vi "AH25_Main.vi"() -> ()   [LabVIEW 2021]
uses:
  GEN_States.ctl
  1375486a-d526-4950-a4e9-ede105372d37.vi
  Sources/Config_Cluster.ctl
  Sources/Data_Cluster.ctl
  <vilib>/Utility/config.llb/NI_LVConfig.lvlib
  Sources/Mode_Enum.ctl
  Sources/Measurement_Cluster.ctl
  Sources/Plotting-Axis.ctl
panel:
  in  "Control Tab":enum32{"General", "Configs"}(tab)
  out "Oven Warning":bool
  out "Capacitance":dbl
  in  "StopM_Button":bool
  in  "Log_Button":bool
  in  "Measure_Button":bool
  out "Globals":bool
  out "AH 2500A":bool
  out "Logging":bool
  out "Measuring":bool
  out "Magnetic Field":dbl
  out "Temperature":dbl
  in  "LoadConfig_Button":bool
  in  "ApplyConfig_Button":bool
  in  "Measure rate (1/s)":i32
  in  "SaveConfig_Button":bool
  in  "Retry_Button":bool
  in  "Config Path (Blank is default)":path
  in  "AH2500 VISA COM":refnum<visa-resource-name>
  in  "Global Temp VAR":refnum<k21>
  in  "Global Mag VAR":refnum<k21>
  in  "Logging Path":path
  in  "Display Tab":enum32{"Program Monitor", "Test Plot"}(tab)
  out "Status":string
  in  "Clear_Button":bool
  in  "Y-Axis":T1
  in  "X-Axis":T1
  out "Test Graph":cluster{"X":dbl, "Y":dbl}[](graph)
  in  "Max Elements":i32=5000
  in  "Exit_Button":bool
  # "Instrument Settings"
  # "Global Var. Settings"
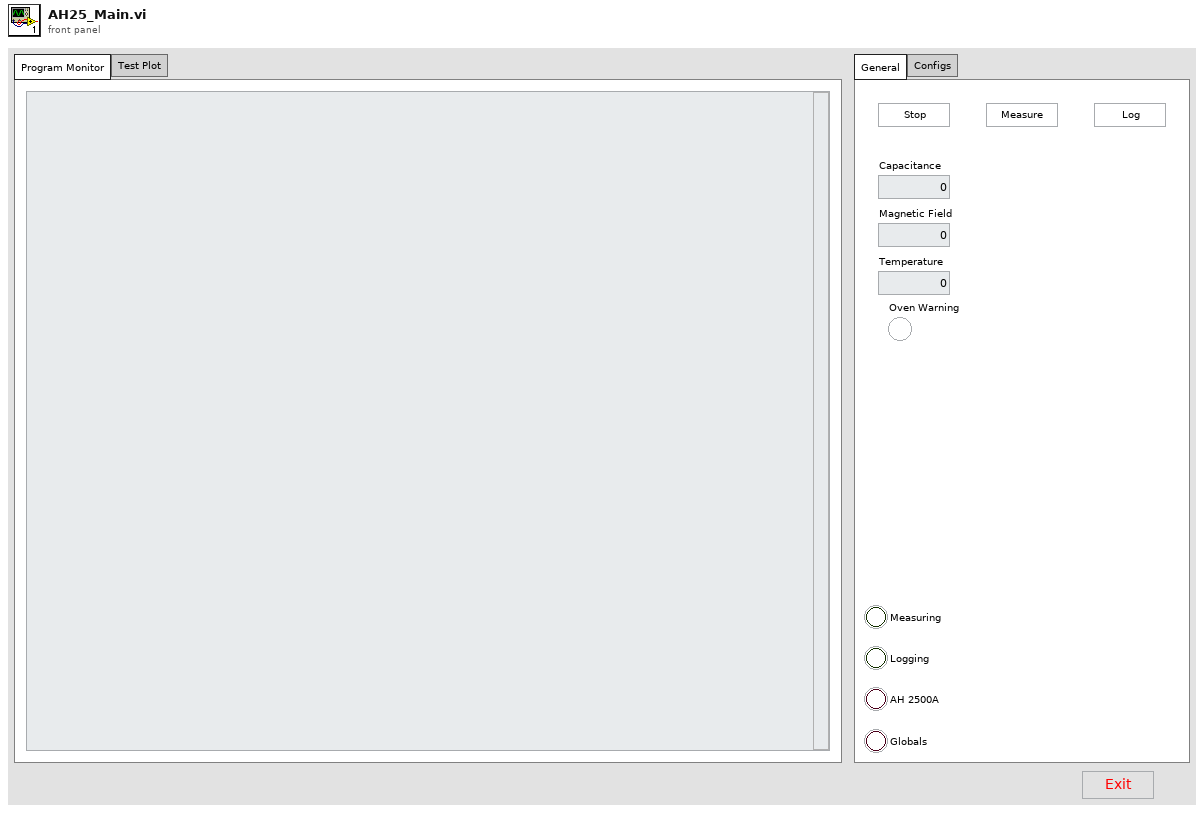
[diagram p1: front panel]
types:
  T1 = typedef "Plotting-Axis.ctl" = enum16{"Time", "Temperature", "MagneticField", "Primary", "Secondary"}
  T2 = typedef "GEN_States.ctl" = enum16{"ClearBuffers", "SwitchToMeas", "SwitchToLog", "SwitchToOff", "Disconnect", "ApplyConfig", "ExitSafe", "RefreshPlotMUnits", "UpdatePlots", "RefreshMUnits", "ChangeOperation", "Read/WriteAll", "RetryComs", "SendProfile", "InitGUI", "RefreshGUI", "ComsFail", "SaveConfig", "Idle", "ProgInit"}
  T3 = typedef "Data_Cluster.ctl" = cluster{"Value":dbl, "GUI Data Cluster":cluster{"SBR":u8}, "Timing":cluster{"Last Operation":dbl}, "Measurements":T4[]}
  T4 = typedef "Measurement_Cluster.ctl" = cluster{"Time Stamp":timestamp, "Cap":dbl, "Temperature":dbl, "MagneticField":dbl}
  T5 = typedef "Config_Cluster.ctl" = cluster{"General":cluster{"Config.ini":path, "Default Logging Path":path}, "Hardware":cluster{"AHC VISA COM":refnum<visa-resource-name>, "Measure Rate (1/s)":i32, "Global T VAR":refnum<k21>, "Global B VAR":refnum<k21>}, "Operation":cluster{"Operation Mode":T6, "Status":string, "NewLog?":bool}}
  T6 = typedef "Mode_Enum.ctl" = enum16{"Logging", "Idle-Off", "Idle"}
  T7 = enum8{"Enabled", "Disabled", "Disabled and Grayed Out"}
  T8 = typedef "NI_LVConfig.lvlib/Config Data RefNum.ctl" = refnum<k1>
  T9 = cluster{"Logging Path":path, "AH2500 VISA COM":refnum<visa-resource-name>, "Measure rate (1/s)":i32, "Global Temp VAR":refnum<k21>, "Global Mag VAR":refnum<k21>}
  T10 = cluster{"Primary Measurement":dbl, "Secondary Measurement":dbl, "T Var":dbl, "B Var":dbl}
  T11 = typedef "GEN_States.ctl" = enum16{"ClearBuffers", "SwitchToMeas", "SwitchToLog", "SwitchToOff", "Disconnect", "ApplyConfig", "ExitSafe", "RefreshPlotMUnits", "UpdatePlots", "RefreshMUnits", "ChangeOperation", "Read/WriteAll", "RetryComs", "SendProfile", "InitGUI", "RefreshGUI", "ComsFail", "LoadProfile", "SaveProfile", "SaveConfig", "Idle", "ProgInit"}
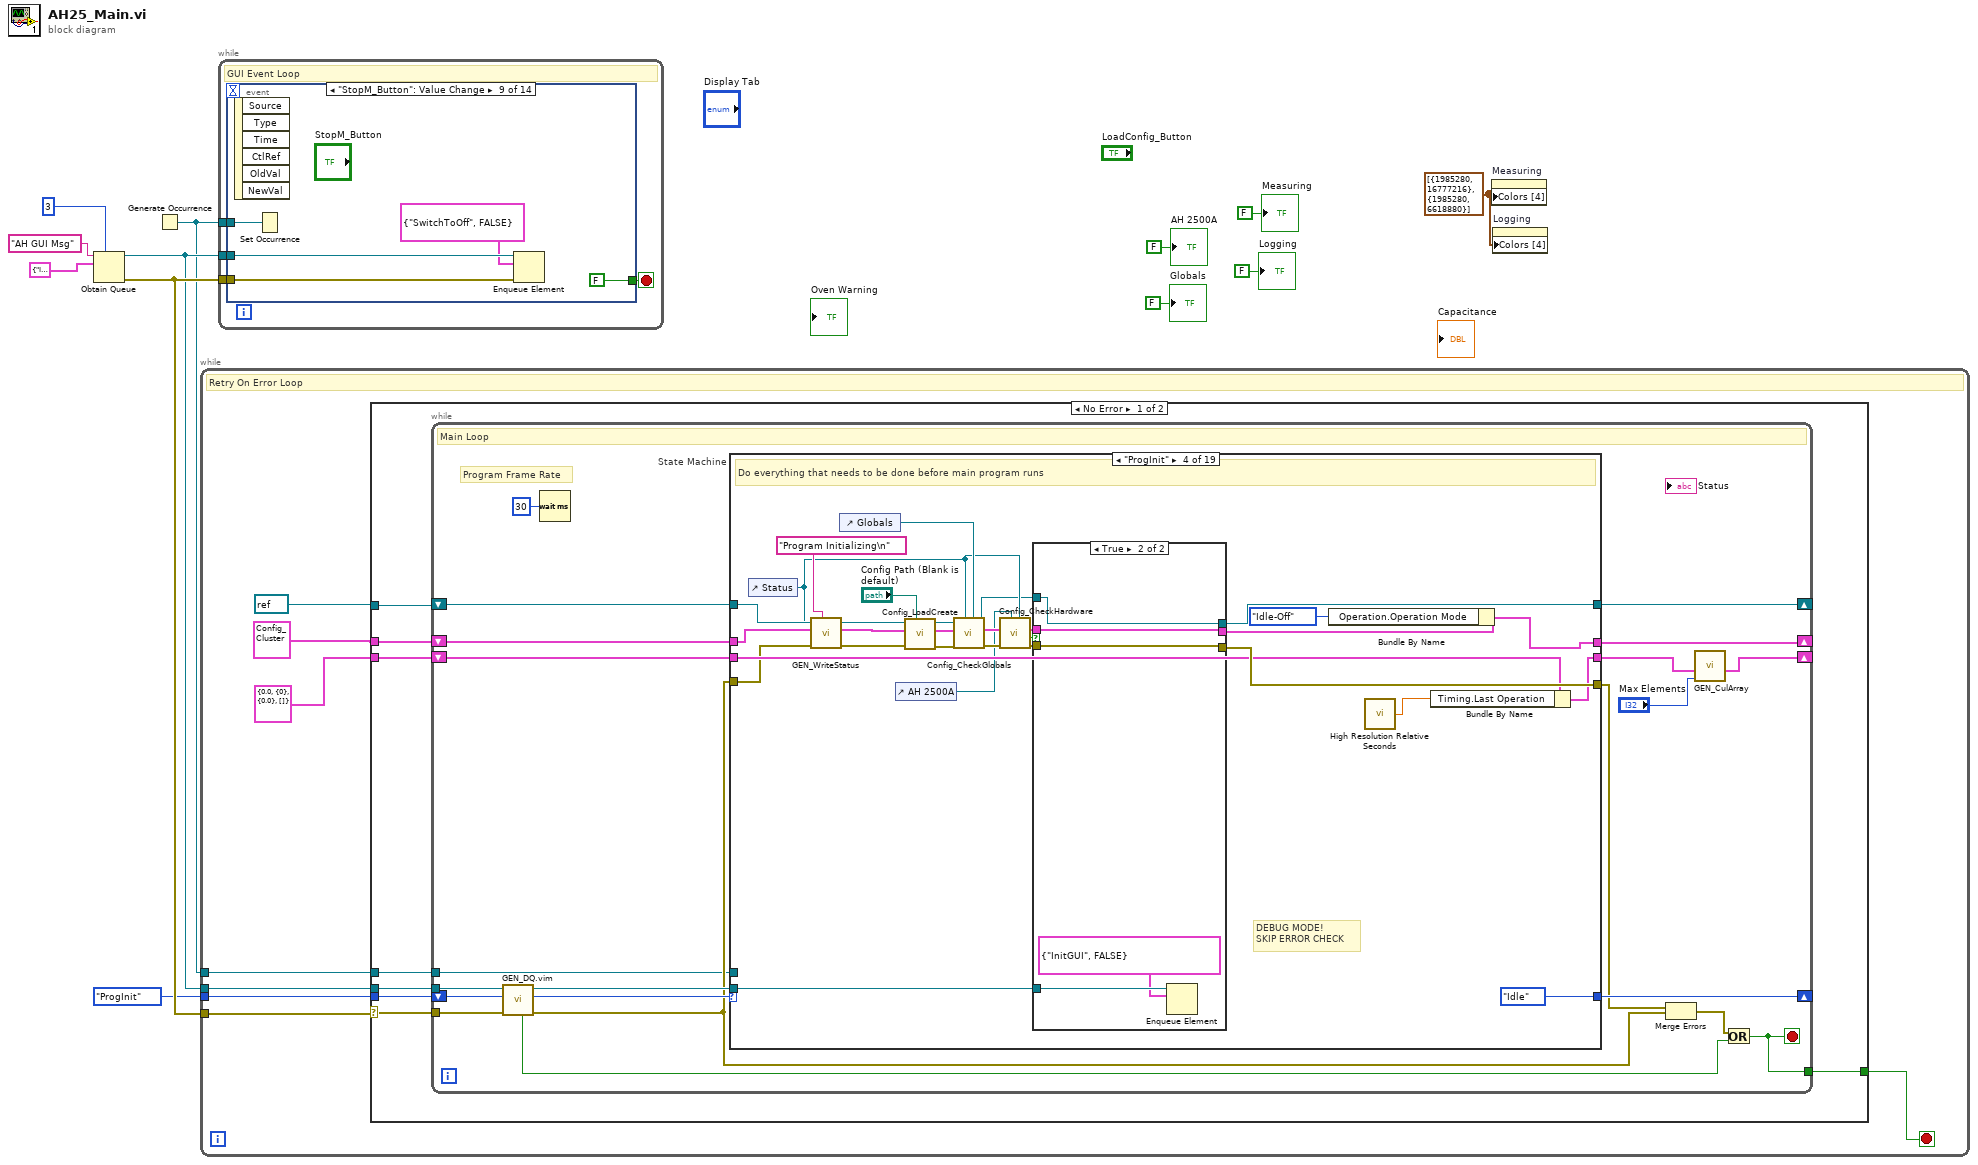
[diagram p0: block diagram]
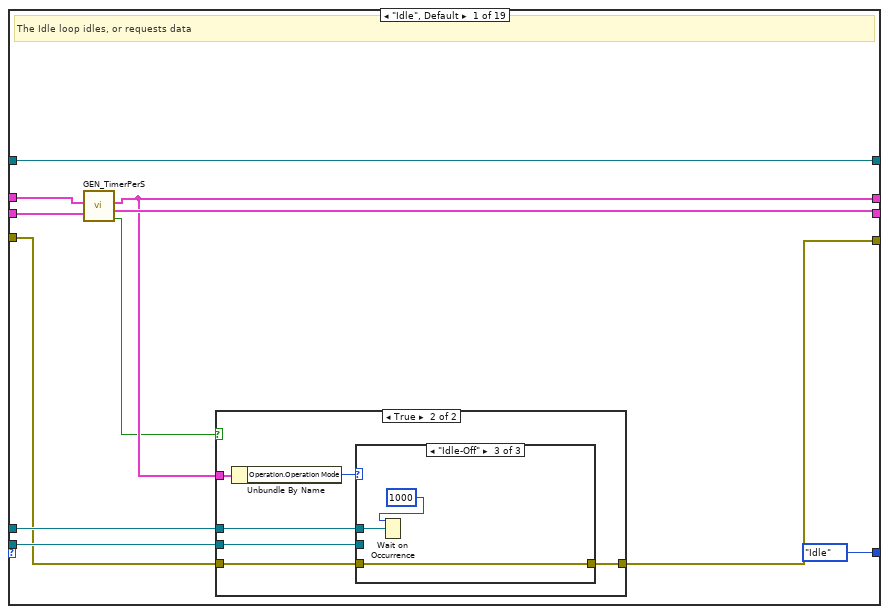
[diagram p2: hidden frame]
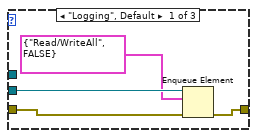
[diagram p4: hidden frame]
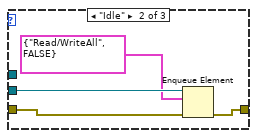
[diagram p5: hidden frame]
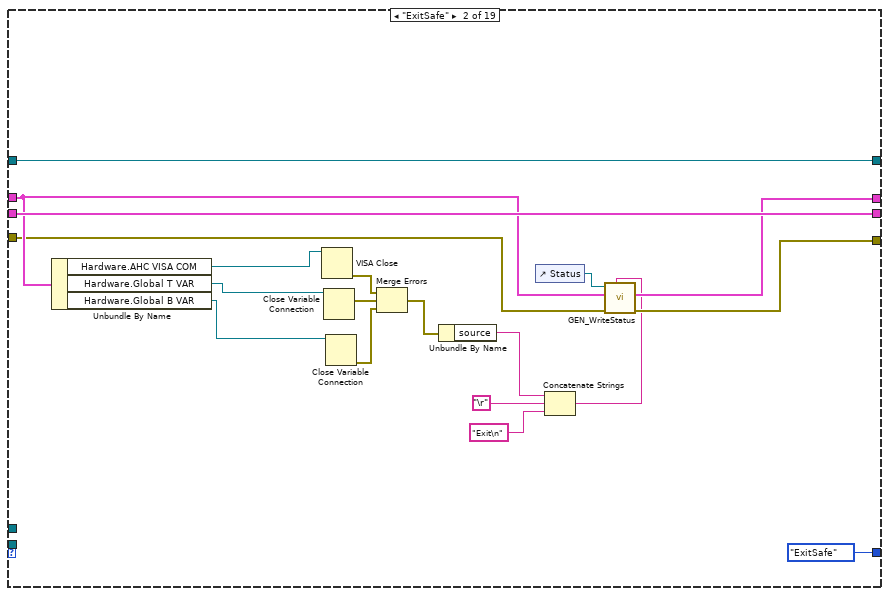
[diagram p6: hidden frame]
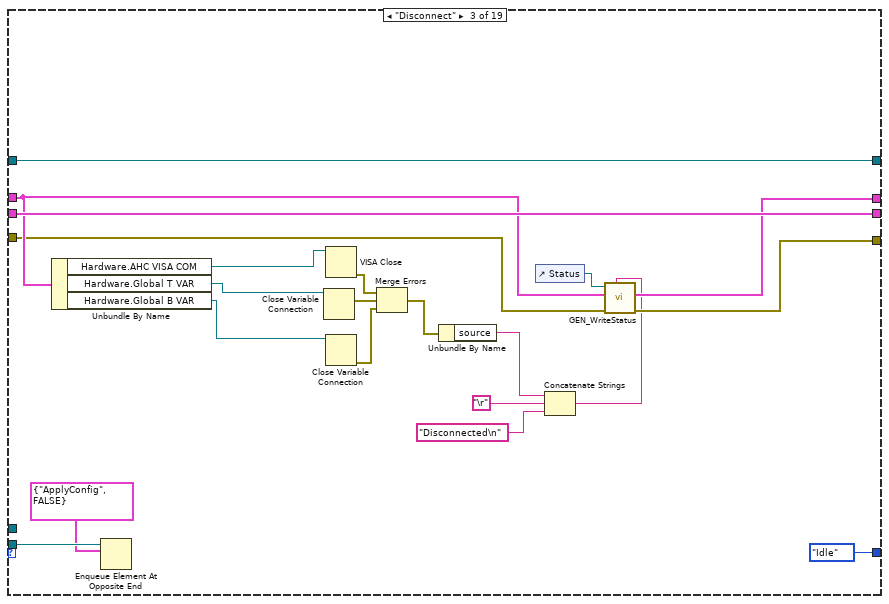
[diagram p7: hidden frame]
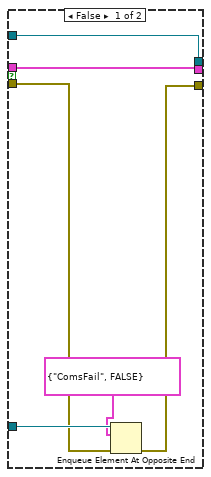
[diagram p8: hidden frame]
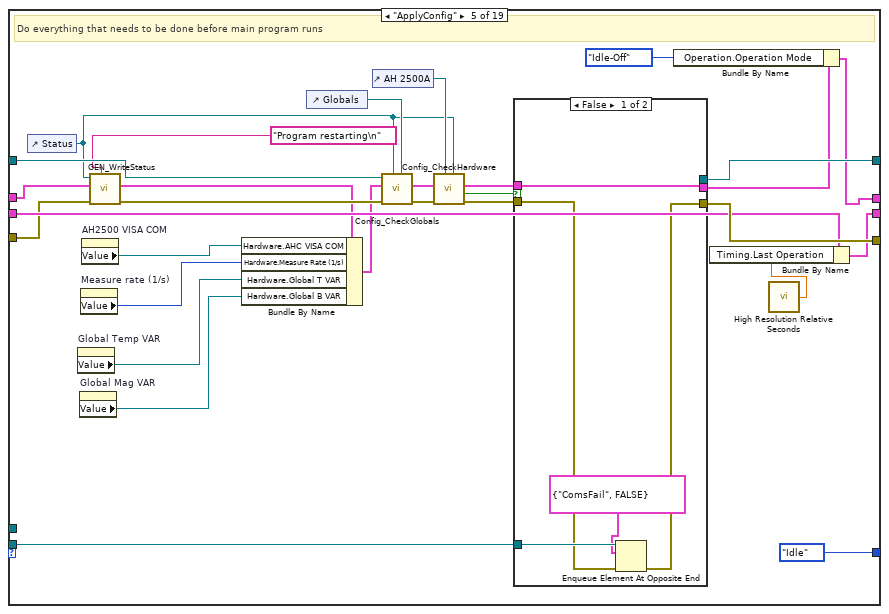
[diagram p9: hidden frame]
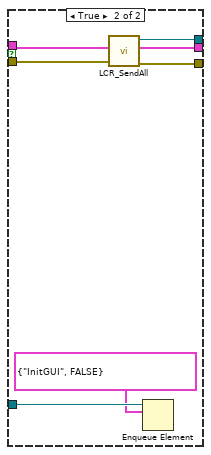
[diagram p10: hidden frame]
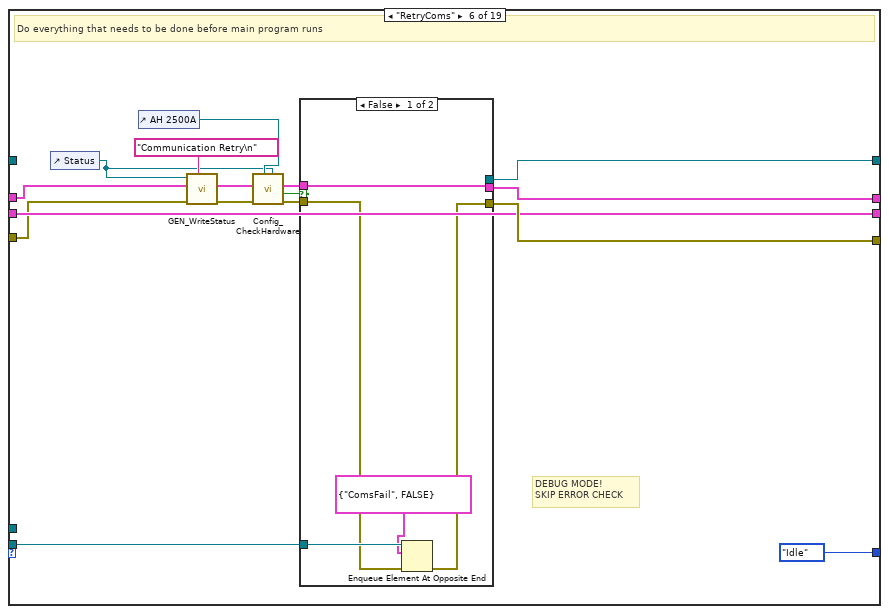
[diagram p11: hidden frame]
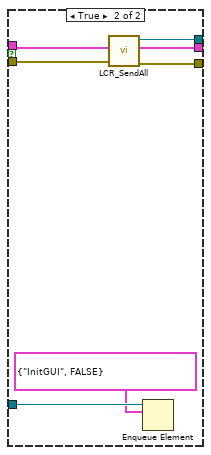
[diagram p12: hidden frame]
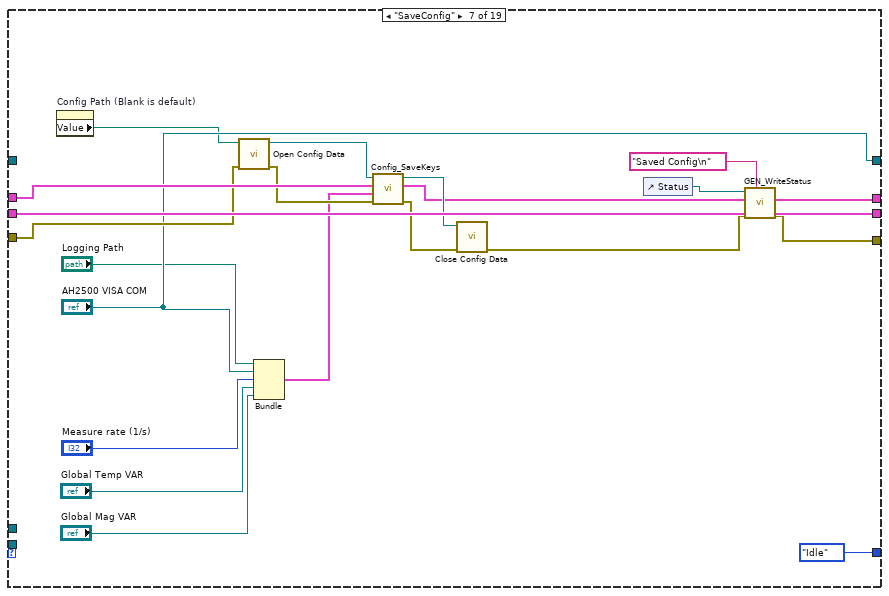
[diagram p13: hidden frame]
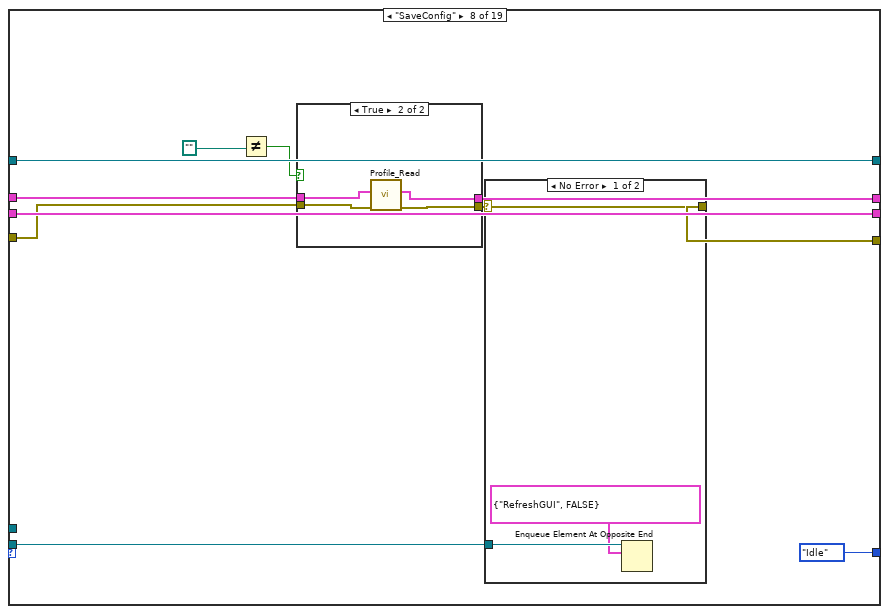
[diagram p14: hidden frame]
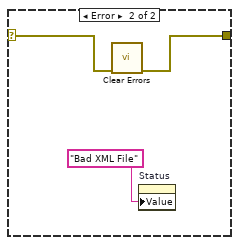
[diagram p15: hidden frame]
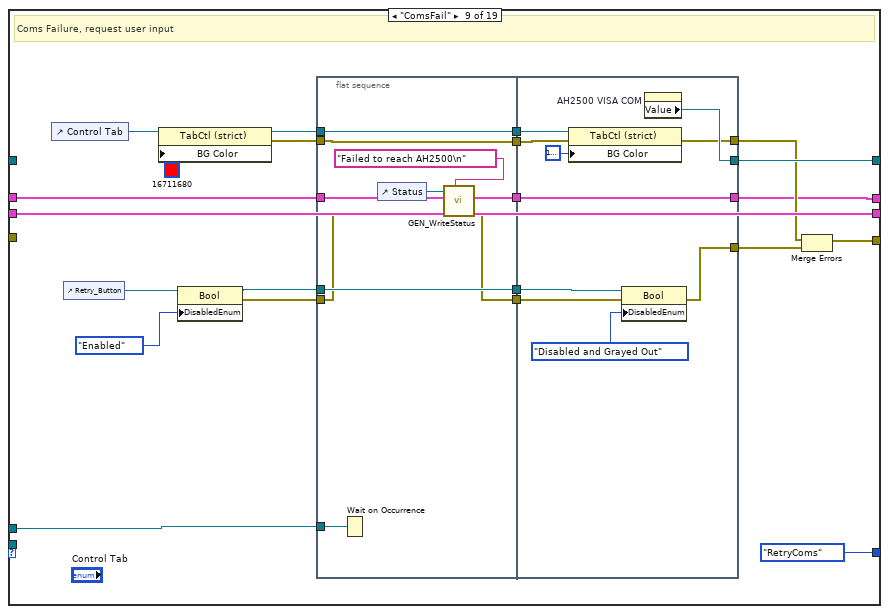
[diagram p17: hidden frame]
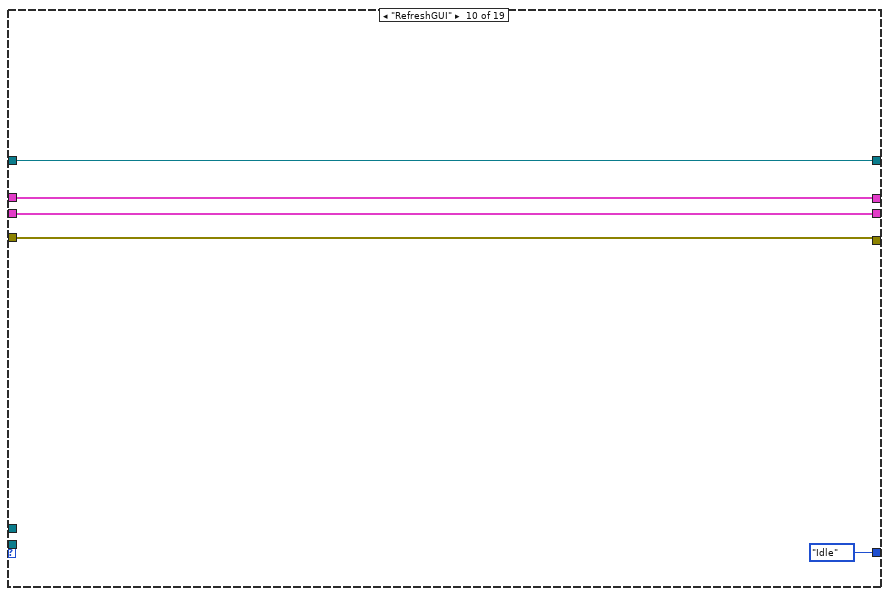
[diagram p18: hidden frame]
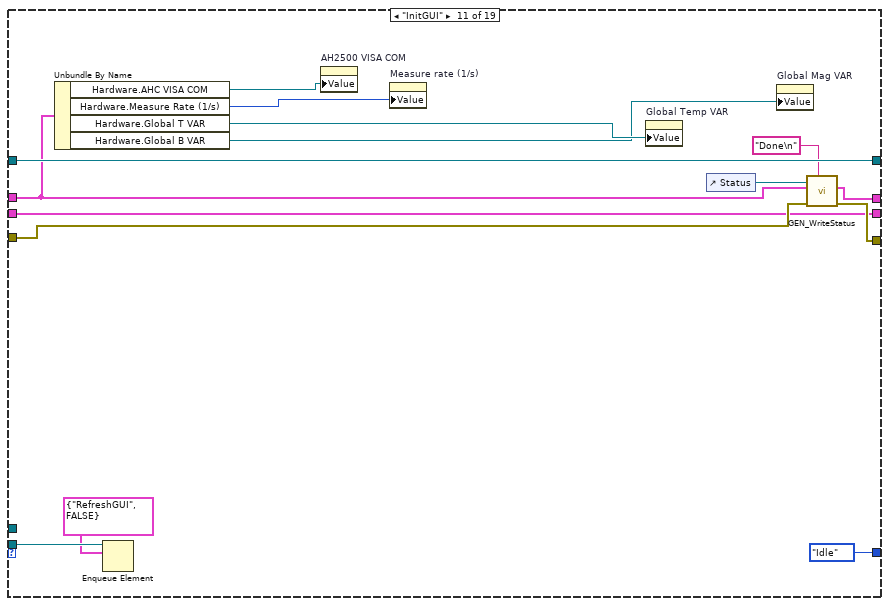
[diagram p19: hidden frame]
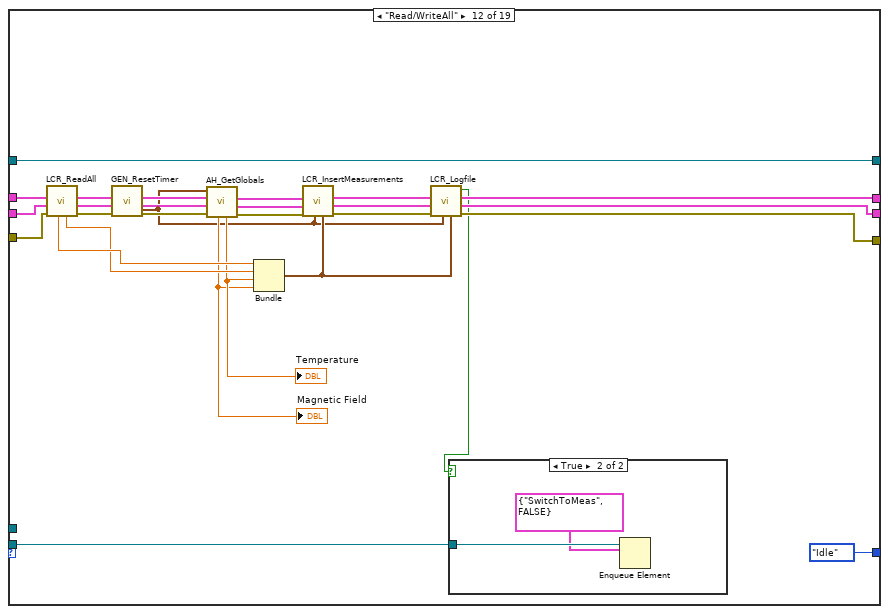
[diagram p20: hidden frame]
diagram:
  w1 = cluster{u32, u32}[] [{1985280, 16777216}, {1985280, 6618880}] ("Colors [4]")
  n1 = Obtain Queue(max queue size (-1, unlimited)=3, name (unnamed)="AH GUI Msg", element data type=cluster{T2, bool} {enum."Idle", TRUE}) -> (queue out=w8:refnum<queue>, error out=w9:errorcluster)  [unwired: 2 in, 1 out]
  n2 = Generate Occurrence() -> (w6:refnum<k4>)
  n3 = while {
    tunnel: w9 -> [w20]
    tunnel: w8 -> [w19]
    tunnel: GEN_States."ProgInit" ("State") -> [w18]
    tunnel: w6 -> [w13]
    stop <- w17 stop-if-true
    # "Retry On Error Loop"
    n4 = case shown="No Error" w20 {
      selector: w20 -> [w28 _]
      tunnel: w19 -> [w27 _]
      tunnel: w18 -> [w26 _]
      tunnel: [w25 TRUE] -> w17
      tunnel: refnum<visa-resource-name> refnum ("LCR VISA COM") -> [w24 _]
      tunnel: T5 {"General"={"Config.ini"=path "", "Default Logging Path"=path ""}, "Hardware"={"AHC VISA COM"="", "Measure Rate (1/s)"=0, "Global T VAR"="", "Global B VAR"=""}, "Operation"={"Operation Mode"=enum."Logging", "Status"="", "NewLog?"=FALSE}} -> [w23 _]
      tunnel: T3 {"Value"=0.0, "GUI Data Cluster"={"SBR"=0}, "Timing"={"Last Operation"=0.0}, "Measurements"=[]} -> [w22 _]
      tunnel: w13 -> [w21 _]
      frame No Error {
        n5 = while {
          tunnel: w28 -> [w48]
          tunnel: w27 -> [w47]
          shift-right: [w40] -> _
          shift-left: w26 -> [w46]
          tunnel: [w42] -> w25
          shift-right: [w39] -> _
          shift-left: w24 -> [w41]
          shift-right: [w36] -> _
          shift-left: w23 -> [w37]
          shift-right: [w30] -> _
          shift-left: w22 -> [w35]
          tunnel: w21 -> [w32]
          stop <- w42 stop-if-true
          # "Program Frame Rate"
          # "Main Loop"
          n6 = call "GEN_DQ.vim"("error in (no error)"=w48, "Variant"=w46, "queue In"=w47) -> ("error out"=w34:errorcluster, "Variant Out"=w45:T2, "queue out"=w38:refnum<queue>, "Exit?"=w43:bool)  [unwired: 5 in]
          n7 = Wait (ms)(milliseconds to wait=u32 30) -> ()  [unwired: 1 out]
          n8 = case "State Machine" shown="\"ProgInit\"" w45 {
            tunnel: w41 -> [w60 w97 w118 w145 w186 _ _ w259 _ w317 w333 w361 w380 w398 w424 w443 w451 w459 w465]
            tunnel: [GEN_States."Idle" ("State") GEN_States."ExitSafe" ("State") GEN_States."Idle" ("State") GEN_States."Idle" ("State") GEN_States."Idle" ("State") GEN_States."Idle" ("State") GEN_States."Idle" ("State") GEN_States."Idle" ("State") GEN_States."RetryComs" ("State") GEN_States."Idle" ("State") GEN_States."Idle" ("State") GEN_States."Idle" ("State") GEN_States."Idle" ("State") GEN_States."Idle" ("State") w410 GEN_States."Idle" ("State") GEN_States."Idle" ("State") GEN_States."Idle" ("State") GEN_States."Idle" ("State")] -> w40
            tunnel: [w60 w97 w118 w140 w181 w209 "AH2500 VISA COM" w259 w286 w317 w333 w361 w380 w398 w424 w443 w451 w459 w465] -> w39
            tunnel: w38 -> [w57 _ w102 w139 w180 w208 _ w249 _ _ w331 w334 _ _ _ _ _ _ _]
            tunnel: w37 -> [w54 w91 w113 w131 w172 w206 w245 w255 w274 w314 w327 w360 w378 w396 w422 w442 w448 w456 w464]
            tunnel: [w51 w90 w112 w132 w173 w210 w235 w254 w273 w314 w326 w355 w375 w393 w411 w442 w448 w456 w464] -> w36
            tunnel: w35 -> [w53 w96 w117 w138 w179 w207 w248 w258 w288 w315 w319 w352 w379 w397 w423 w438 w449 w457 w462]
            tunnel: [w52 w96 w117 w137 w178 w207 w248 w258 w288 w315 w319 w349 w379 w397 w423 w437 w449 w457 w461] -> w31
            tunnel: w34 -> [w56 w89 w111 w129 w171 w203 w244 w256 _ w316 w324 w359 w370 w388 w416 w436 w447 w455 w463]
            tunnel: [w55 w88 w110 w141 w182 w211 w231 w250 w277 w316 w323 w356 w369 w387 w415 w436 w447 w455 w463] -> w33
            tunnel: w32 -> [w58 _ _ _ _ _ _ _ w287 _ _ _ _ _ _ _ _ _ _]
            frame "Idle", Default {
              # "The Idle loop idles, or requests data"
              n9 = call "GEN_TimerPerS.vi"("Data_In"=w53, "Config_In"=w54) -> ("Time"=w50:bool, "Data_In 2"=w52:T3, "Config_In 2"=w51:T5)  [unwired: 7 in]
              n10 = case shown="True" w50 {
                tunnel: w58 -> [_ w66]
                tunnel: w57 -> [_ w65]
                tunnel: w56 -> [w61 w64]
                tunnel: [w61 w63] -> w55
                tunnel: w51 -> [_ w62]
                frame False {
                }
                frame True {
                  n11 = Unbundle By Name(w62) -> ("Operation.Operation Mode"=w67:T6)
                  n12 = case shown="\"Idle-Off\"" w67 {
                    tunnel: w66 -> [_ _ w78]
                    tunnel: w65 -> [w71 w75 _]
                    tunnel: w64 -> [w70 w74 w77]
                    tunnel: [w68 w72 w77] -> w63
                    frame "Logging", Default {
                      n13 = Enqueue Element(queue=w71, element=cluster{T2, bool} {enum."Read/WriteAll", FALSE}, error in (no error)=w70) -> (error out=w68:errorcluster)  [unwired: 1 in, 2 out]
                    }
                    frame "Idle" {
                      n14 = Enqueue Element(queue=w75, element=cluster{T2, bool} {enum."Read/WriteAll", FALSE}, error in (no error)=w74) -> (error out=w72:errorcluster)  [unwired: 1 in, 2 out]
                    }
                    frame "Idle-Off" {
                      n15 = Wait on Occurrence(2:w78, 3:1000 ("ms timeout (-1)")) -> ()  [unwired: 1 in, 1 out]
                    }
                  }
                }
              }
            }
            frame "ExitSafe" {
              n16 = Unbundle By Name(w91) -> ("Hardware.AHC VISA COM"=w80:refnum<visa-resource-name>, "Hardware.Global T VAR"=w94:refnum<k21>, "Hardware.Global B VAR"=w93:refnum<k21>)
              n17 = VISA Close(VISA resource name=w80) -> (error out=w79:errorcluster)  [unwired: 1 in]
              n18 = Close Variable Connection(11:w94) -> (0:w86:errorcluster)  [unwired: 1 in]
              n19 = Close Variable Connection(11:w93) -> (0:w87:errorcluster)  [unwired: 1 in]
              n20 = Merge Errors(w79, w86, w87) -> (w85:errorcluster)
              n21 = Unbundle By Name(w85) -> ("source"=w83:string)
              n22 = control-ref of="Status"() -> (w92:refnum<vi>)
              n23 = Concatenate Strings(w83, "\r", "Exit\n" ("string")) -> (w84:string)
              n24 = call "GEN_WriteStatus.vi"("Input String"=w84, "error in (no error)"=w89, "Config_Cluster"=w91, "Status Ref"=w92) -> ("error out"=w88:errorcluster, "Config_Cluster Out"=w90:T5)  [unwired: 6 in]
            }
            frame "Disconnect" {
              n25 = Unbundle By Name(w113) -> ("Hardware.AHC VISA COM"=w99:refnum<visa-resource-name>, "Hardware.Global T VAR"=w116:refnum<k21>, "Hardware.Global B VAR"=w115:refnum<k21>)
              n26 = Enqueue Element At Opposite End(queue=w102, element=cluster{T2, bool} {enum."ApplyConfig", FALSE}) -> ()  [unwired: 2 in, 3 out]
              n27 = Close Variable Connection(11:w116) -> (0:w108:errorcluster)  [unwired: 1 in]
              n28 = VISA Close(VISA resource name=w99) -> (error out=w98:errorcluster)  [unwired: 1 in]
              n29 = Close Variable Connection(11:w115) -> (0:w109:errorcluster)  [unwired: 1 in]
              n30 = Merge Errors(w98, w108, w109) -> (w107:errorcluster)
              n31 = Unbundle By Name(w107) -> ("source"=w105:string)
              n32 = control-ref of="Status"() -> (w114:refnum<vi>)
              n33 = Concatenate Strings(w105, "\r", "Disconnected\n" ("string")) -> (w106:string)
              n34 = call "GEN_WriteStatus.vi"("Input String"=w106, "error in (no error)"=w111, "Config_Cluster"=w113, "Status Ref"=w114) -> ("error out"=w110:errorcluster, "Config_Cluster Out"=w112:T5)  [unwired: 6 in]
            }
            frame "ProgInit" {
              # "DEBUG MODE!\nSKIP ERROR CHECK"
              # "Do everything that needs to be done before main program runs"
              n35 = control-ref of="Status"() -> (w120:refnum<vi>)
              n36 = call "GEN_WriteStatus.vi"("Input String"="Program Initializing\n" ("Status"), "error in (no error)"=w129, "Config_Cluster"=w131, "Status Ref"=w120) -> ("error out"=w128:errorcluster, "Config_Cluster Out"=w130:T5)  [unwired: 6 in]
              n37 = control-ref of="Globals"() -> (w122:refnum<vi>)
              n38 = control-ref of="AH 2500A"() -> (w121:refnum<vi>)
              n39 = call "Config_LoadCreate.vi"("Config In"="Config Path (Blank is default)", "error In"=w128, "Configuration Cluster"=w130, "AH VISA COM"=w145) -> ("error out"=w124:errorcluster, "Configuration Cluster Out"=w125:T5, "AHC VISA COM Out"=w127:refnum<visa-resource-name>)  [unwired: 5 in]
              n40 = call "Config_CheckGlobals.vi"("GlobalsLED Ref"=w122, "Status Ref"=w120, "error in (no error)"=w124, "Config Cluster"=w125, "VISA resource name"=w127) -> ("error out"=w123:errorcluster, "Config Cluster Out"=w126:T5, "VISA resource name out"=w119:refnum<visa-resource-name>)  [unwired: 4 in]
              n41 = call "Config_CheckHardware.vi"("Status Ref"=w120, "HM 8119"=w121, "error in (no error)"=w123, "Config Cluster"=w126) -> ("error out"=w143:errorcluster, "Connected?"=w144:bool, "Config Cluster Out"=w142:T5)  [unwired: 5 in]
              n42 = case shown="True" w144 {
                tunnel: w143 -> [w149 w157]
                tunnel: w142 -> [w152 w158]
                tunnel: w119 -> [w153 w154]
                tunnel: [w153 w154] -> w140
                tunnel: [w152 w158] -> w135
                tunnel: [w148 w157] -> w141
                tunnel: w139 -> [w151 w156]
                frame False {
                  n43 = Enqueue Element At Opposite End(queue=w151, element=cluster{T2, bool} {enum."ComsFail", FALSE}, error in (no error)=w149) -> (error out=w148:errorcluster)  [unwired: 1 in, 2 out]
                }
                frame True {
                  n44 = Enqueue Element(queue=w156, element=cluster{T2, bool} {enum."InitGUI", FALSE}) -> ()  [unwired: 2 in, 3 out]
                }
              }
              n45 = Bundle By Name(cluster=w135, "Operation.Operation Mode"=Mode_Enum."Idle-Off") -> (w132:T5)
              n46 = call <vilib>:"High Resolution Relative Seconds.vi"() -> ("relative seconds"=w136:dbl)
              n47 = Bundle By Name(cluster=w138, "Timing.Last Operation"=w136) -> (w137:T3)
            }
            frame "ApplyConfig" {
              # "Do everything that needs to be done before main program runs"
              n48 = control-ref of="Status"() -> (w160:refnum<vi>)
              n49 = property on="Global Temp VAR" class="Variable (strict)"() -> ("Value"=w164:refnum<k21>)  [unwired: 2 in, 2 out]
              n50 = property on="Global Mag VAR" class="Variable (strict)"() -> ("Value"=w163:refnum<k21>)  [unwired: 2 in, 2 out]
              n51 = property on="Measure rate (1/s)" class="DigNum (strict)"() -> ("Value"=w165:i32)  [unwired: 2 in, 2 out]
              n52 = property on="AH2500 VISA COM" class="VISAName"() -> ("Value"=w159:refnum<visa-resource-name>)  [unwired: 2 in, 2 out]
              n53 = call "GEN_WriteStatus.vi"("Input String"="Program restarting\n" ("Status"), "error in (no error)"=w171, "Config_Cluster"=w172, "Status Ref"=w160) -> ("error out"=w170:errorcluster, "Config_Cluster Out"=w167:T5)  [unwired: 6 in]
              n54 = Bundle By Name(cluster=w167, "Hardware.AHC VISA COM"=w159, "Hardware.Measure Rate (1/s)"=w165, "Hardware.Global T VAR"=w164, "Hardware.Global B VAR"=w163) -> (w166:T5)
              n55 = control-ref of="Globals"() -> (w162:refnum<vi>)
              n56 = control-ref of="AH 2500A"() -> (w161:refnum<vi>)
              n57 = call "Config_CheckGlobals.vi"("GlobalsLED Ref"=w162, "Status Ref"=w160, "error in (no error)"=w170, "Config Cluster"=w166, "VISA resource name"=w186) -> ("error out"=w168:errorcluster, "Config Cluster Out"=w169:T5)  [unwired: 4 in, 1 out]
              n58 = call "Config_CheckHardware.vi"("Status Ref"=w160, "HM 8119"=w161, "error in (no error)"=w168, "Config Cluster"=w169) -> ("error out"=w184:errorcluster, "Connected?"=w185:bool, "Config Cluster Out"=w183:T5)  [unwired: 5 in]
              n59 = case shown="False" w185 {
                tunnel: w184 -> [w189 w198]
                tunnel: w183 -> [w192 w199]
                tunnel: [_ w197] -> w181
                tunnel: [w192 w196] -> w176
                tunnel: [w188 w195] -> w182
                tunnel: w180 -> [w191 w194]
                frame False {
                  n60 = Enqueue Element At Opposite End(queue=w191, element=cluster{T2, bool} {enum."ComsFail", FALSE}, error in (no error)=w189) -> (error out=w188:errorcluster)  [unwired: 1 in, 2 out]
                }
                frame True {
                  n61 = call "LCR_SendAll.vi"("error in (no error)"=w198, "Configuration Cluster"=w199) -> ("error out"=w195:errorcluster, "Configuration Cluster Out"=w196:T5, "VISA resource name out"=w197:refnum<visa-resource-name>)  [unwired: 7 in]
                  n62 = Enqueue Element(queue=w194, element=cluster{T2, bool} {enum."InitGUI", FALSE}) -> ()  [unwired: 2 in, 3 out]
                }
              }
              n63 = Bundle By Name(cluster=w176, "Operation.Operation Mode"=Mode_Enum."Idle-Off") -> (w173:T5)
              n64 = call <vilib>:"High Resolution Relative Seconds.vi"() -> ("relative seconds"=w177:dbl)
              n65 = Bundle By Name(cluster=w179, "Timing.Last Operation"=w177) -> (w178:T3)
            }
            frame "RetryComs" {
              # "DEBUG MODE!\nSKIP ERROR CHECK"
              # "Do everything that needs to be done before main program runs"
              n66 = control-ref of="Status"() -> (w200:refnum<vi>)
              n67 = control-ref of="AH 2500A"() -> (w201:refnum<vi>)
              n68 = call "GEN_WriteStatus.vi"("Input String"="Communication Retry\n", "error in (no error)"=w203, "Config_Cluster"=w206, "Status Ref"=w200) -> ("error out"=w202:errorcluster, "Config_Cluster Out"=w205:T5)  [unwired: 6 in]
              n69 = call "Config_CheckHardware.vi"("Status Ref"=w200, "HM 8119"=w201, "error in (no error)"=w202, "Config Cluster"=w205) -> ("error out"=w213:errorcluster, "Connected?"=w214:bool, "Config Cluster Out"=w212:T5)  [unwired: 5 in]
              n70 = case shown="False" w214 {
                tunnel: w213 -> [w217 w226]
                tunnel: w212 -> [w220 w227]
                tunnel: [_ w225] -> w209
                tunnel: [w220 w224] -> w210
                tunnel: [w216 w223] -> w211
                tunnel: w208 -> [w219 w222]
                frame False {
                  n71 = Enqueue Element At Opposite End(queue=w219, element=cluster{T2, bool} {enum."ComsFail", FALSE}, error in (no error)=w217) -> (error out=w216:errorcluster)  [unwired: 1 in, 2 out]
                }
                frame True {
                  n72 = call "LCR_SendAll.vi"("error in (no error)"=w226, "Configuration Cluster"=w227) -> ("error out"=w223:errorcluster, "Configuration Cluster Out"=w224:T5, "VISA resource name out"=w225:refnum<visa-resource-name>)  [unwired: 7 in]
                  n73 = Enqueue Element(queue=w222, element=cluster{T2, bool} {enum."InitGUI", FALSE}) -> ()  [unwired: 2 in, 3 out]
                }
              }
            }
            frame "SaveConfig" {
              n74 = property on="Config Path (Blank is default)" class="Path"() -> ("Value"=w238:path)  [unwired: 2 in, 2 out]
              n75 = call <vilib>:"Open Config Data.vi"("error in (no error)"=w244, "configuration file path"=w238) -> ("error out"=w243:errorcluster, "refnum"=w242:T8)  [unwired: 7 in, 1 out]
              n76 = Bundle("Logging Path"="Logging Path", "AH2500 VISA COM"="AH2500 VISA COM", "Measure rate (1/s)"="Measure rate (1/s)", "Global Temp VAR"="Global Temp VAR", "Global Mag VAR"="Global Mag VAR") -> (w228:T9)  [unwired: 1 in]
              n77 = call "Config_SaveKeys.vi"("error in (no error)"=w243, "Settings In"=w228, "Configuration Cluster"=w245, "Config In"=w242) -> ("error out"=w240:errorcluster, "output cluster"=w236:T5, "refnum out"=w241:T8)  [unwired: 5 in]
              n78 = call <vilib>:"Close Config Data.vi"("error in (no error)"=w240, "refnum"=w241) -> ("error out"=w232:errorcluster)  [unwired: 8 in, 1 out]
              n79 = control-ref of="Status"() -> (w233:refnum<vi>)
              n80 = call "GEN_WriteStatus.vi"("Input String"="Saved Config\n", "error in (no error)"=w232, "Config_Cluster"=w236, "Status Ref"=w233) -> ("error out"=w231:errorcluster, "Config_Cluster Out"=w235:T5)  [unwired: 6 in]
            }
            frame "SaveConfig" {
              n81 = Not Equal?(y=path "") -> (x != y?=w252:bool)  [unwired: 1 in]
              n82 = case shown="True" w252 {
                tunnel: w256 -> [w266 w271]
                tunnel: w255 -> [w267 w270]
                tunnel: [w266 w269] -> w251
                tunnel: [w267 w268] -> w254
                frame False {
                }
                frame True {
                  n83 = call "Profile_Read.vi"("error in (no error)"=w271, "Configuration Cluster"=w270) -> ("error out"=w269:errorcluster, "Configuration Cluster Out"=w268:T5)  [unwired: 8 in]
                }
              }
              n84 = case shown="No Error" w251 {
                selector: w251 -> [w262 w265]
                tunnel: [w262 w264] -> w250
                tunnel: w249 -> [w261 _]
                frame No Error {
                  n85 = Enqueue Element At Opposite End(queue=w261, element=cluster{T2, bool} {enum."RefreshGUI", FALSE}) -> ()  [unwired: 2 in, 3 out]
                }
                frame Error {
                  n86 = call <vilib>:"Clear Errors.vi"("error in (no error)"=w265) -> ("error out"=w264:errorcluster)  [unwired: 5 in, 1 out]
                  n87 = property on="Status" class="Str"("Value"="Bad XML File" ("Status")) -> ()  [unwired: 2 in, 2 out]
                }
              }
            }
            frame "ComsFail" {
              # "Coms Failure, request user input"
              n88 = control-ref of="Control Tab"() -> (w293:refnum<vi>)
              n89 = control-ref of="Retry_Button"() -> (w292:refnum<vi>)
              n90 = property on="Property Node" class="TabCtl (strict)"(reference=w293, "BG Color"=u32 16711680 ("Colors:BG Color")) -> (reference out=w284:refnum<vi>, error out=w283:errorcluster)  [unwired: 1 in]
              n91 = property class="Bool"(reference=w292, "DisabledEnum"=T7."Enabled" ("Disabled")) -> (reference out=w280:refnum<vi>, error out=w279:errorcluster)  [unwired: 1 in]
              n92 = flat-sequence {
                tunnel: w287 -> [w303]
                tunnel: [w302] -> w285
                tunnel: w284 -> [w302]
                tunnel: w283 -> [w301]
                tunnel: [w301] -> w282
                tunnel: [w300] -> w281
                tunnel: w280 -> [w300]
                tunnel: w279 -> [w296]
                tunnel: [w295] -> w278
                tunnel: w274 -> [w299]
                tunnel: [w298] -> w272
                tunnel: [w313] -> w286
                tunnel: w285 -> [w312]
                tunnel: w282 -> [w311]
                tunnel: w281 -> [w310]
                tunnel: w278 -> [w309]
                tunnel: [w307] -> w276
                tunnel: [w306] -> w275
                tunnel: [w304] -> w273
                tunnel: w272 -> [w304]
                frame #0 {
                  n93 = Wait on Occurrence(2:w303) -> ()  [unwired: 2 in, 1 out]
                  n94 = control-ref of="Status"() -> (w294:refnum<vi>)
                  n95 = call "GEN_WriteStatus.vi"("Input String"="Failed to reach AH2500\n", "error in (no error)"=w296, "Config_Cluster"=w299, "Status Ref"=w294) -> ("error out"=w295:errorcluster, "Config_Cluster Out"=w298:T5)  [unwired: 6 in]
                }
                frame #1 {
                  n96 = property class="TabCtl (strict)"(reference=w312, error in=w311, "BG Color"=u32 16777226 ("Colors:BG Color")) -> (error out=w307:errorcluster)  [unwired: 1 out]
                  n97 = property class="Bool"(reference=w310, error in=w309, "DisabledEnum"=T7."Disabled and Grayed Out" ("Disabled")) -> (error out=w306:errorcluster)  [unwired: 1 out]
                  n98 = property on="AH2500 VISA COM" class="VISAName"() -> ("Value"=w313:refnum<visa-resource-name>)  [unwired: 2 in, 2 out]
                }
              }
              n99 = Merge Errors(w276, w275) -> (w277:errorcluster)
            }
            frame "RefreshGUI" {
            }
            frame "InitGUI" {
              n100 = Unbundle By Name(w327) -> ("Hardware.AHC VISA COM"=w329:refnum<visa-resource-name>, "Hardware.Measure Rate (1/s)"=w328:i32, "Hardware.Global T VAR"=w321:refnum<k21>, "Hardware.Global B VAR"=w320:refnum<k21>)
              n101 = Enqueue Element(queue=w331, element=cluster{T2, bool} {enum."RefreshGUI", FALSE}) -> ()  [unwired: 2 in, 3 out]
              n102 = property on="AH2500 VISA COM" class="VISAName"("Value"=w329) -> ()  [unwired: 2 in, 2 out]
              n103 = property on="Measure rate (1/s)" class="DigNum (strict)"("Value"=w328) -> ()  [unwired: 2 in, 2 out]
              n104 = property on="Global Temp VAR" class="Variable (strict)"("Value"=w321) -> ()  [unwired: 2 in, 2 out]
              n105 = control-ref of="Status"() -> (w322:refnum<vi>)
              n106 = property on="Global Mag VAR" class="Variable (strict)"("Value"=w320) -> ()  [unwired: 2 in, 2 out]
              n107 = call "GEN_WriteStatus.vi"("Input String"="Done\n", "error in (no error)"=w324, "Config_Cluster"=w327, "Status Ref"=w322) -> ("error out"=w323:errorcluster, "Config_Cluster Out"=w326:T5)  [unwired: 6 in]
            }
            frame "Read/WriteAll" {
              n108 = call "LCR_ReadAll.vi"("error in (no error)"=w359, "Data_In"=w352, "Configuration Cluster"=w360) -> ("error out"=w358:errorcluster, "Data_Out"=w351:T3, "Configuration Cluster 2"=w354:T5, "Secondary Measurement"=w347:dbl, "Primary Measurement"=w348:dbl)  [unwired: 4 in]
              n109 = call "GEN_ResetTimer.vi"("error in (no error)"=w358, "Data_In"=w351, "Cluster IN"=w354) -> ("error out"=w343:errorcluster, "Data_In 2"=w344:T3, "Cluster OUT"=w345:T5, "TimeStamp"=w337:timestamp)  [unwired: 5 in]
              n110 = call "AH_GetGlobals.vi"("error in (no error)"=w343, "Data_In"=w344, "Cluster IN"=w345, "Start Stamp"=w337) -> ("error out"=w340:errorcluster, "Data_Out"=w341:T3, "Cluster OUT"=w342:T5, "T Var"=w339:dbl, "B Var"=w338:dbl)  [unwired: 1 in, 2 out]
              "Temperature" <- w339
              "Magnetic Field" <- w338
              n111 = Bundle("Primary Measurement"=w348, "Secondary Measurement"=w347, "T Var"=w339, "B Var"=w338) -> (w346:T10)  [unwired: 1 in]
              n112 = call "LCR_InsertMeasurements.vi"("Data Cluster"=w346, "TimeStamp"=w337, "error in (no error)"=w340, "Data_IN"=w341, "Cluster IN"=w342) -> ("error out"=w336:errorcluster, "Data_OUT"=w350:T3, "Cluster OUT"=w353:T5)  [unwired: 4 in]
              n113 = call "LCR_Logfile.vi"("Data Cluster"=w346, "Time Stamp"=w337, "error in"=w336, "Data_In"=w350, "Config_In"=w353) -> ("error out"=w356:errorcluster, "Data_Out"=w349:T3, "Config_Out"=w355:T5, "File Failure"=w335:bool)  [unwired: 3 in]
              n114 = case shown="True" w335 {
                tunnel: w334 -> [w363 w365]
                frame False {
                  n115 = Enqueue Element(queue=w363, element=cluster{T2, bool} {enum."UpdatePlots", FALSE}) -> ()  [unwired: 2 in, 3 out]
                }
                frame True {
                  n116 = Enqueue Element(queue=w365, element=cluster{T2, bool} {enum."SwitchToMeas", FALSE}) -> ()  [unwired: 2 in, 3 out]
                }
              }
            }
            frame "SwitchToOff" {
              w374 = Mode_Enum."Idle-Off" ("Operation.Operation Mode")
              n117 = Bundle By Name(cluster=w378, "Operation.Operation Mode"=w374) -> (w376:T5)
              n118 = case shown="\"Logging\", Default" w374 {
                tunnel: ["Measure and logging\n" "Off\n" "Measure only\n"] -> w373
                frame "Logging", Default {
                }
                frame "Idle-Off" {
                }
                frame "Idle" {
                }
              }
              n119 = control-ref of="Status"() -> (w368:refnum<vi>)
              n120 = Concatenate Strings("Changed Mode to: " ("string"), w373) -> (w371:string)
              n121 = call "GEN_WriteStatus.vi"("Input String"=w371, "error in (no error)"=w370, "Config_Cluster"=w376, "Status Ref"=w368) -> ("error out"=w369:errorcluster, "Config_Cluster Out"=w375:T5)  [unwired: 6 in]
              n122 = property on="Measuring" class="Bool (strict)"("Value"=FALSE ("Measuring")) -> ()  [unwired: 2 in, 2 out]
              n123 = property on="Logging" class="Bool (strict)"("Value"=FALSE ("Logging")) -> ()  [unwired: 2 in, 2 out]
            }
            frame "SwitchToMeas" {
              w392 = Mode_Enum."Idle" ("Operation.Operation Mode")
              n124 = Bundle By Name(cluster=w396, "Operation.Operation Mode"=w392) -> (w394:T5)
              n125 = case shown="\"Idle\"" w392 {
                tunnel: ["Measure and logging\n" "Off\n" "Measure only\n"] -> w391
                frame "Logging", Default {
                }
                frame "Idle-Off" {
                }
                frame "Idle" {
                }
              }
              n126 = control-ref of="Status"() -> (w386:refnum<vi>)
              n127 = Concatenate Strings("Changed Mode to: " ("string"), w391) -> (w389:string)
              n128 = call "GEN_WriteStatus.vi"("Input String"=w389, "error in (no error)"=w388, "Config_Cluster"=w394, "Status Ref"=w386) -> ("error out"=w387:errorcluster, "Config_Cluster Out"=w393:T5)  [unwired: 6 in]
              n129 = property on="Measuring" class="Bool (strict)"("Value"=TRUE ("Measuring")) -> ()  [unwired: 2 in, 2 out]
              n130 = property on="Logging" class="Bool (strict)"("Value"=FALSE ("Logging")) -> ()  [unwired: 2 in, 2 out]
            }
            frame "SwitchToLog" {
              w420 = Mode_Enum."Logging" ("Operation.Operation Mode")
              n131 = call "File Dialog"("prompt"="Where do you want to log measurements?", "default name"="LogFile.csv", "pattern (all files)"="*.csv", "pattern label"="CSV file") -> ("selected path"=w409:path, "cancelled"=w413:bool)  [unwired: 8 in, 2 out]
              n132 = Bundle By Name(cluster=w422, "Operation.Operation Mode"=w420, "Operation.NewLog?"=TRUE) -> (w421:T5)
              n133 = case shown="\"Logging\", Default" w420 {
                tunnel: ["Measure and logging\n" "Off\n" "Measure only\n"] -> w419
                frame "Logging", Default {
                }
                frame "Idle-Off" {
                }
                frame "Idle" {
                }
              }
              n134 = control-ref of="Status"() -> (w414:refnum<vi>)
              n135 = Concatenate Strings("Changed Mode to: " ("string"), w419) -> (w417:string)
              n136 = property on="Logging" class="Bool (strict)"("Value"=TRUE ("Logging")) -> ()  [unwired: 2 in, 2 out]
              n137 = property on="Measuring" class="Bool (strict)"("Value"=TRUE ("Measuring")) -> ()  [unwired: 2 in, 2 out]
              n138 = call "GEN_WriteStatus.vi"("Input String"=w417, "error in (no error)"=w416, "Config_Cluster"=w421, "Status Ref"=w414) -> ("error out"=w415:errorcluster, "Config_Cluster Out"=w412:T5)  [unwired: 6 in]
              n139 = case shown="False" w413 {
                tunnel: w412 -> [w427 w429]
                tunnel: [w426 w429] -> w411
                tunnel: [GEN_States."RefreshMUnits" ("State") GEN_States."SwitchToMeas" ("State")] -> w410
                tunnel: w409 -> [w425 _]
                frame False {
                  n140 = Bundle By Name(cluster=w427, "General.Default Logging Path"=w425) -> (w426:T5)
                }
                frame True {
                }
              }
            }
            frame "UpdatePlots" {
              n141 = control-ref of="Test Graph"() -> (w441:refnum<vi>)
              n142 = call "LCR_PlotHelper.vi"("Y-Axis"="Y-Axis", "X-Axis"="X-Axis", "Data_IN"=w438, "Graph REF"=w441) -> ("Graph Out"=→"Test Graph":cluster{"Variant X":dbl, "Variant Y":dbl}[], "Data_Out"=w437:T3)  [unwired: 6 in]
            }
            frame "RefreshPlotMUnits" {
              n143 = control-ref of="Test Graph"() -> (w446:refnum<vi>)
              n144 = property on="Y-Axis" class="Enum (strict)"() -> ("Value"=w444:T1)  [unwired: 2 in, 2 out]
              n145 = property on="X-Axis" class="Enum (strict)"() -> ("Value"=w445:T1)  [unwired: 2 in, 2 out]
              n146 = call "LCR_PlotNamer.vi"("Y-Axis"=w444, "X-Axis"=w445, "Graph Ref In"=w446) -> ()  [unwired: 9 in]
            }
            frame "RefreshMUnits" {
              n147 = control-ref of="Test Graph"() -> (w454:refnum<vi>)
              n148 = property on="Y-Axis" class="Enum (strict)"() -> ("Value"=w452:T1)  [unwired: 2 in, 2 out]
              n149 = property on="X-Axis" class="Enum (strict)"() -> ("Value"=w453:T1)  [unwired: 2 in, 2 out]
              n150 = call "LCR_PlotNamer.vi"("Y-Axis"=w452, "X-Axis"=w453, "Graph Ref In"=w454) -> ()  [unwired: 9 in]
            }
            frame "ClearBuffers" {
              n151 = in-place {
                n152 = in-place-cluster #1(w462) -> ("Measurements"=w467:T4[])
                n153 = Array Size(array=w467) -> (size(s)=w466:i32)
                n154 = Delete From Array(array=w467, length=w466, index=0) -> (array with subset deleted=w469:T4[])  [unwired: 1 out]
                n155 = in-place-cluster #1("Measurements"=w469) -> (w461:T3)
              }
            }
          }
          n156 = Merge Errors(w33, w34) -> (w44:errorcluster)
          n157 = call "GEN_CulArray.vi"("Max Values"="Max Elements", "Data_Cluster"=w31) -> ("Data_Cluster Out"=w30:T3)  [unwired: 9 in]
          n158 = Or(x=w44, y=w43) -> (x .or. y?=w42:bool)
        }
      }
      frame Error {
      }
    }
  }
  n159 = while {
    tunnel: w8 -> [w474]
    tunnel: w9 -> [w473]
    tunnel: w6 -> [w471]
    stop <- w472 stop-if-true
    # "GUI Event Loop"
    n160 = event shown="[8] \"StopM_Button\": Value Change" {
      selector: _ -> [_ _ _ _ _ _ _ _ _ _ _ _ _ _]
      dyn-events: _ -> [_ _ _ _ _ _ _ _ _ _ _ _ _ _]
      timeout: _ -> [_ _ _ _ _ _ _ _ _ _ _ _ _ _]
      tunnel: w474 -> [_ w479 w484 w488 w493 w497 w502 w507 w512 w517 w522 w527 w532 w537]
      tunnel: w473 -> [_ w478 w483 w487 w492 w496 w501 w506 w511 w516 w521 w526 w531 w536]
      tunnel: [_ TRUE FALSE FALSE FALSE FALSE FALSE FALSE FALSE FALSE FALSE FALSE FALSE FALSE] -> w472
      tunnel: w471 -> [_ w475 w480 w485 w489 w494 w498 w503 w508 w513 w518 w523 w528 w533]
      event Timeout {
        n161 = event-data() -> ()  [unwired: 1 in, 3 out]
      }
      event "Exit_Button": Value Change {
        n162 = event-data() -> ()  [unwired: 1 in, 6 out]
        n163 = Set Occurrence(w475) -> ()
        n164 = Enqueue Element At Opposite End(queue=w479, element=cluster{T2, bool} {enum."ExitSafe", TRUE}, error in (no error)=w478) -> ()  [unwired: 1 in, 3 out]
      }
      event "Retry_Button": Value Change {
        n165 = event-data() -> ()  [unwired: 1 in, 6 out]
        n166 = Set Occurrence(w480) -> ()
        n167 = Enqueue Element At Opposite End(queue=w484, element=cluster{T2, bool} {enum."RetryComs", FALSE}, error in (no error)=w483) -> ()  [unwired: 1 in, 3 out]
      }
      event #3 (no event record) {
        (unwired) cluster{T11, bool} {enum."LoadProfile", FALSE} ("element")
        n168 = event-data() -> ()  [unwired: 1 in, 6 out]
        n169 = Set Occurrence(w485) -> ()
        n170 = Enqueue Element(queue=w488, error in (no error)=w487) -> ()  [unwired: 2 in, 3 out]
      }
      event "ApplyConfig_Button": Value Change {
        n171 = event-data() -> ()  [unwired: 1 in, 6 out]
        n172 = Set Occurrence(w489) -> ()
        n173 = Enqueue Element(queue=w493, element=cluster{T2, bool} {enum."Disconnect", FALSE}, error in (no error)=w492) -> ()  [unwired: 1 in, 3 out]
      }
      event #5 (no event record) {
        (unwired) cluster{T11, bool} {enum."SaveProfile", FALSE} ("element")
        n174 = event-data() -> ()  [unwired: 1 in, 6 out]
        n175 = Set Occurrence(w494) -> ()
        n176 = Enqueue Element(queue=w497, error in (no error)=w496) -> ()  [unwired: 2 in, 3 out]
      }
      event "SaveConfig_Button": Value Change {
        n177 = event-data() -> ()  [unwired: 1 in, 6 out]
        n178 = Set Occurrence(w498) -> ()
        n179 = Enqueue Element(queue=w502, element=cluster{T2, bool} {enum."SaveConfig", FALSE}, error in (no error)=w501) -> ()  [unwired: 1 in, 3 out]
      }
      event #7 (no event record) {
        n180 = event-data() -> ()  [unwired: 1 in, 6 out]
        n181 = Set Occurrence(w503) -> ()
        n182 = Enqueue Element(queue=w507, element=cluster{T2, bool} {enum."SendProfile", FALSE}, error in (no error)=w506) -> ()  [unwired: 1 in, 3 out]
      }
      event "StopM_Button": Value Change {
        n183 = event-data() -> ()  [unwired: 1 in, 6 out]
        n184 = Set Occurrence(w508) -> ()
        n185 = Enqueue Element(queue=w512, element=cluster{T2, bool} {enum."SwitchToOff", FALSE}, error in (no error)=w511) -> ()  [unwired: 1 in, 3 out]
      }
      event "Measure_Button": Value Change {
        n186 = event-data() -> ()  [unwired: 1 in, 6 out]
        n187 = Set Occurrence(w513) -> ()
        n188 = Enqueue Element(queue=w517, element=cluster{T2, bool} {enum."SwitchToMeas", FALSE}, error in (no error)=w516) -> ()  [unwired: 1 in, 3 out]
      }
      event "Log_Button": Value Change {
        n189 = event-data() -> ()  [unwired: 1 in, 6 out]
        n190 = Set Occurrence(w518) -> ()
        n191 = Enqueue Element(queue=w522, element=cluster{T2, bool} {enum."SwitchToLog", FALSE}, error in (no error)=w521) -> ()  [unwired: 1 in, 3 out]
      }
      event #11 (no event record) {
        n192 = event-data() -> ()  [unwired: 1 in, 6 out]
        n193 = Set Occurrence(w523) -> ()
        n194 = Enqueue Element(queue=w527, element=cluster{T2, bool} {enum."RefreshMUnits", FALSE}, error in (no error)=w526) -> ()  [unwired: 1 in, 3 out]
      }
      event "Clear_Button": Value Change {
        n195 = event-data() -> ()  [unwired: 1 in, 6 out]
        n196 = Set Occurrence(w528) -> ()
        n197 = Enqueue Element(queue=w532, element=cluster{T2, bool} {enum."ClearBuffers", FALSE}, error in (no error)=w531) -> ()  [unwired: 1 in, 3 out]
      }
      event Value Change {
        n198 = event-data() -> ()  [unwired: 1 in, 6 out]
        n199 = Set Occurrence(w533) -> ()
        n200 = Enqueue Element(queue=w537, element=cluster{T2, bool} {enum."RefreshPlotMUnits", FALSE}, error in (no error)=w536) -> ()  [unwired: 1 in, 3 out]
      }
    }
  }
  n201 = property on="Measuring" class="Bool (strict)"("Colors [4]"=w1) -> ()  [unwired: 2 in, 2 out]
  n202 = property on="Logging" class="Bool (strict)"("Colors [4]"=w1) -> ()  [unwired: 2 in, 2 out]
  "Globals" <- FALSE ("Globals")
  "AH 2500A" <- FALSE ("HM 8118")
  "Logging" <- FALSE ("Logging")
  "Measuring" <- FALSE ("Measuring")
